vi "Station.vi"(8 "station #":i32, 11 "command":T3) -> (3 "status":T2)   [LabVIEW 2019]
uses:
  <extravilib>/ChannelInstances/MessengerM-t'Command.ctl'/))Channel.ctl
  Command.ctl
  <extravilib>/ChannelInstances/Messenger-c(i32,t'Status.ctl')/))Channel.ctl
  Status.ctl
  74d80a09-c140-2b42-92c2-15952b1630e7.vi
  <extravilib>/ChannelInstances/Messenger-c(i32,t'Status.ctl')/Write With Abort.vi
  <extravilib>/ChannelInstances/MessengerM-t'Command.ctl'/Read With Abort.vi
  <resource>/Channels/Messenger/Write With Abort.vi
  <extravilib>/ChannelInstances/Messenger-c(i32,t'Status.ctl')/Wrapper.lvclass
  C:/Program Files (x86)/National Instruments/LabVIEW 2019/vi.lib/ChannelSupport/Channel Message/Channel Message.lvclass
  <extravilib>/ChannelInstances/Messenger-c(i32,t'Status.ctl')/Wrap.vi
  <resource>/Channels/Messenger/Endpoint.vi
  <extravilib>/ChannelInstances/MessengerM-t'Command.ctl'/Endpoint.vi
  <extravilib>/ChannelInstances/MessengerM-t'Command.ctl'.lvlib
  <extravilib>/ChannelInstances/Messenger-c(i32,t'Status.ctl').lvlib
panel:
  out "status":T1 items=["exited", "off", "active", "standby", "error"]
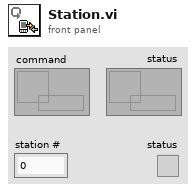
[diagram p1: front panel]
types:
  T1 = typedef "Status.ctl" = u16
  T2 = typedef "Messenger-c(i32,t'Status.ctl').lvlib/))Channel.ctl" = refnum<queue>
  T3 = typedef "MessengerM-t'Command.ctl'.lvlib/))Channel.ctl" = refnum<queue>
  T4 = enum16{"stop", "pause", "error", "exit", "default"}
  T5 = enum16{"_Quit_", "Off", "Active", "Standby", "Error", "Exit"}
  T6 = enum16{"_Quit_", "Off", "Active", "Standby", "Error", "Exit"}[]
  T7 = typedef "Command.ctl" = enum16{"start", "stop", "pause", "resume", "reset", "exit"}
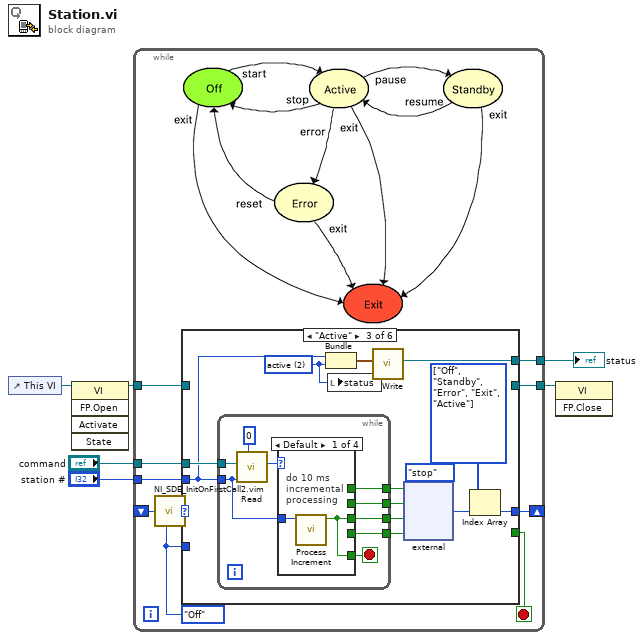
[diagram p0: block diagram]
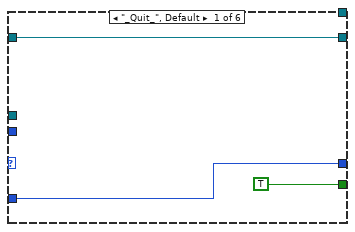
[diagram p2: hidden frame]
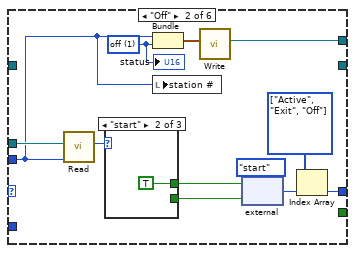
[diagram p3: hidden frame]
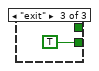
[diagram p5: hidden frame]
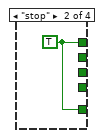
[diagram p6: hidden frame]
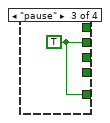
[diagram p7: hidden frame]
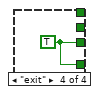
[diagram p8: hidden frame]
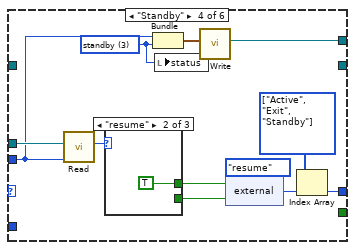
[diagram p9: hidden frame]
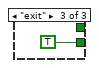
[diagram p11: hidden frame]
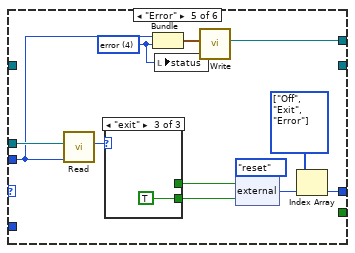
[diagram p12: hidden frame]
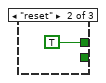
[diagram p14: hidden frame]
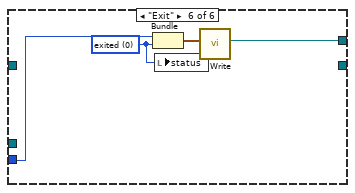
[diagram p15: hidden frame]
diagram:
  n1 = control-ref of="This VI"() -> (w3:refnum<vi>)
  n2 = invoke class="VI" method="FP.Open"(reference=w3) -> (reference out=w2:refnum<vi>)  [unwired: 4 in, 4 out]
  n3 = while {
    shift-right: [w13] -> _
    shift-left: _ -> [w16]
    tunnel: "command" -> [w11]
    tunnel: "station #" -> [w10]
    tunnel: [w9] -> w4
    tunnel: w2 -> [w7]
    tunnel: [w8] -> w1
    stop <- w14 stop-if-true
    w12 = T5."Off"
    n4 = call "NI_SDE_InitOnFirstCall2.vim"("input"=w16, "master enum"=w12) -> ("output enum"=w15:T5)  [unwired: 1 in]
    n5 = case shown="\"Active\"" w15 {
      tunnel: [TRUE _ _ _ _ _] -> w14
      tunnel: [w18 w31 w55 w92 w115 _] -> w13
      tunnel: w12 -> [w18 _ _ _ _ _]
      tunnel: w11 -> [_ w27 w49 w85 w110 _]
      tunnel: w10 -> [_ w20 w48 w84 w106 w128]
      tunnel: [_ w26 w50 w87 w105 w129] -> w9
      tunnel: [w17 _ _ _ _ _] -> w8
      tunnel: w7 -> [w17 _ _ _ _ _]
      frame "_Quit_", Default {
      }
      frame "Off" {
        w21 = T1 1 items=["exited", "off", "active", "standby", "error"] ("status")
        w28 = T6 [enum."Active", enum."Exit", enum."Off"] items=["_Quit_", "Off", "Active", "Standby", "Error", "Exit"]
        n6 = call <extravilib>:"Read.vi"("subchannel (0)"=w20, "channel"=w27) -> ("element"=w22:T7)  [unwired: 5 in, 4 out]
        n7 = case shown="\"start\"" w22 {
          tunnel: [_ TRUE _] -> w24
          tunnel: [_ _ TRUE] -> w23
          frame Default {
          }
          frame "start" {
          }
          frame "exit" {
          }
        }
        n8 = Bundle("station #"=w20, "status"=w21) -> (w25:cluster{"station #":i32, "status":T1})  [unwired: 1 in]
        n9 = local write "station #"(w20) -> ()
        n10 = call <extravilib>:"Write.vi"("element"=w25) -> ("channel"=w26:T2)  [unwired: 8 in, 2 out]
        n11 = external ("First Transition")(enum16{"start", "exit", "default"}."start", w24, w23) -> (w30:enum16{"start", "exit", "default"})
        n12 = Index Array(array=w28, index=w30) -> (element=w31:T5)
        "status" <- w21
      }
      frame "Active" {
        w43 = T1 2 items=["exited", "off", "active", "standby", "error"] ("status")
        w52 = T6 [enum."Off", enum."Standby", enum."Error", enum."Exit", enum."Active"] items=["_Quit_", "Off", "Active", "Standby", "Error", "Exit"]
        n13 = while {
          tunnel: w49 -> [w64]
          tunnel: w48 -> [w56]
          tunnel: [w61] -> w47
          tunnel: [w60] -> w46
          tunnel: [w59] -> w45
          tunnel: [w58] -> w44
          stop <- w57 stop-if-true
          n14 = call <extravilib>:"Read.vi"("timeout in ms (-1)"=0, "subchannel (0)"=w56, "channel"=w64) -> ("element"=w62:T7)  [unwired: 4 in, 4 out]
          n15 = case shown="Default" w62 {
            tunnel: [_ w67 _ _] -> w61
            tunnel: [_ _ w68 _] -> w60
            tunnel: [_ _ _ w69] -> w59
            tunnel: [w66 _ _ _] -> w58
            tunnel: [w66 w67 w68 w69] -> w57
            tunnel: w56 -> [w65 _ _ _]
            frame Default {
              # "do 10 ms\nincremental\nprocessing"
              n16 = call "Process Increment.vi"("station #"=w65) -> ("error"=w66:bool)  [unwired: 10 in]
            }
            frame "stop" {
              w67 = TRUE
            }
            frame "pause" {
              w68 = TRUE
            }
            frame "exit" {
              w69 = TRUE
            }
          }
        }
        n17 = Bundle("station #"=w48, "status"=w43) -> (w51:cluster{"station #":i32, "status":T1})  [unwired: 1 in]
        n18 = local write "status"(w43) -> ()
        n19 = call <extravilib>:"Write.vi"("element"=w51) -> ("channel"=w50:T2)  [unwired: 8 in, 2 out]
        n20 = external ("First Transition")(T4."stop", w47, w46, w44, w45) -> (w54:T4)
        n21 = Index Array(array=w52, index=w54) -> (element=w55:T5)
      }
      frame "Standby" {
        w81 = T1 3 items=["exited", "off", "active", "standby", "error"] ("status")
        w89 = T6 [enum."Active", enum."Exit", enum."Standby"] items=["_Quit_", "Off", "Active", "Standby", "Error", "Exit"]
        n22 = call <extravilib>:"Read.vi"("subchannel (0)"=w84, "channel"=w85) -> ("element"=w86:T7)  [unwired: 5 in, 4 out]
        n23 = case shown="\"resume\"" w86 {
          tunnel: [_ TRUE _] -> w83
          tunnel: [_ _ TRUE] -> w82
          frame Default {
          }
          frame "resume" {
          }
          frame "exit" {
          }
        }
        n24 = Bundle("station #"=w84, "status"=w81) -> (w88:cluster{"station #":i32, "status":T1})  [unwired: 1 in]
        n25 = local write "status"(w81) -> ()
        n26 = call <extravilib>:"Write.vi"("element"=w88) -> ("channel"=w87:T2)  [unwired: 8 in, 2 out]
        n27 = external ("First Transition")(enum16{"resume", "exit", "default"}."resume", w83, w82) -> (w91:enum16{"resume", "exit", "default"})
        n28 = Index Array(array=w89, index=w91) -> (element=w92:T5)
      }
      frame "Error" {
        w104 = T1 4 items=["exited", "off", "active", "standby", "error"] ("status")
        w112 = T6 [enum."Off", enum."Exit", enum."Error"] items=["_Quit_", "Off", "Active", "Standby", "Error", "Exit"]
        n29 = call <extravilib>:"Read.vi"("subchannel (0)"=w106, "channel"=w110) -> ("element"=w111:T7)  [unwired: 5 in, 4 out]
        n30 = case shown="\"exit\"" w111 {
          tunnel: [_ TRUE _] -> w109
          tunnel: [_ _ TRUE] -> w108
          frame Default {
          }
          frame "reset" {
          }
          frame "exit" {
          }
        }
        n31 = Bundle("station #"=w106, "status"=w104) -> (w107:cluster{"station #":i32, "status":T1})  [unwired: 1 in]
        n32 = local write "status"(w104) -> ()
        n33 = call <extravilib>:"Write.vi"("element"=w107) -> ("channel"=w105:T2)  [unwired: 8 in, 2 out]
        n34 = external ("First Transition")(enum16{"reset", "exit", "default"}."reset", w109, w108) -> (w114:enum16{"reset", "exit", "default"})
        n35 = Index Array(array=w112, index=w114) -> (element=w115:T5)
      }
      frame "Exit" {
        w127 = T1 0 items=["exited", "off", "active", "standby", "error"] ("status")
        n36 = Bundle("station #"=w128, "status"=w127) -> (w130:cluster{"station #":i32, "status":T1})  [unwired: 1 in]
        n37 = local write "status"(w127) -> ()
        n38 = call <extravilib>:"Write.vi"("element"=w130) -> ("channel"=w129:T2)  [unwired: 8 in, 2 out]
      }
    }
  }
  "status" <- w4
  n39 = invoke class="VI" method="FP.Close"(reference=w1) -> ()  [unwired: 2 in, 3 out]
